vi "PhotonPipelineMetadata_GetLatency.vi"(11 "PhotonPipelineMetadata":T1={"CaptureTimestampMicros"=-1, "PublishTimestampMicros"=-1, "SequenceID"=-1, "TimeSinceLastPong"=9999999999}) -> (3 "Latency_ms":dbl)   [LabVIEW 2019, in "PhotonVisionLib.lvlib"]
doc: "Returns the time between image capture and publish to NT\n\nInputs:\n - PipelineMetadata -- Parsed PipelineMetadata cluster.\n\nOutputs:\n - Latency_ms -- Latency between cature and publish (milliseconds)"
uses:
  TypeDef/PhotonPipelineMetadataType.ctl
  PhotonVisionLib.lvlib
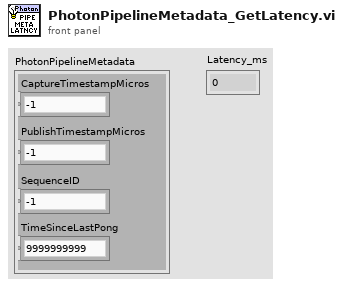
[diagram p1: front panel]
types:
  T1 = typedef "PhotonVisionLib.lvlib/PhotonPipelineMetadataType.ctl" = cluster{"CaptureTimestampMicros":i64, "PublishTimestampMicros":i64, "SequenceID":i64, "TimeSinceLastPong":i64}
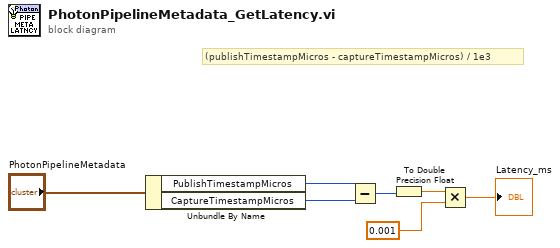
[diagram p0: block diagram]
diagram:
  # "(publishTimestampMicros - captureTimestampMicros) / 1e3"
  n1 = Unbundle By Name("PhotonPipelineMetadata") -> ("PublishTimestampMicros"=w6:i64, "CaptureTimestampMicros"=w5:i64)
  n2 = Subtract(x=w6, y=w5) -> (x-y=w4:i64)
  n3 = To Double Precision Float(number=w4) -> (double precision float=w3:dbl)
  n4 = Multiply(x=w3, y=0.001) -> (x*y=→"Latency_ms":dbl)
